vi "Monitor Tool Page.vi"(8 "error in (no error)":errorcluster, 11 "Node Ptr":T1 format="%.0x") -> (0 "error out":errorcluster)   [LabVIEW 2023, in "J1939 Addon System Explorer.lvlib"]
uses:
  J1939 Addon System Explorer.lvlib
  <vilib>/NI VeriStand/Custom Device API/Custom Device Item Ref.ctl
  Addon Shared/SubVIs/Constants.vi
  <vilib>/NI VeriStand/Custom Device API/Custom Device API.lvlib
  Addon Shared/J1939 Addon Shared.lvlib
panel:
  in  "Force SA":bool
  in  "Include DA":bool
  in  "Settings":cluster{"Section Name":string}={"Section Name"="J1939 Monitor Tool Settings"}
  in  "J1939 Name":u64 format="%.0x"
  in  "J1939 Network Address":u8 format="%.0x"
  in  "SHDocVw.IWebBrowser2":refnum<k7>(container)
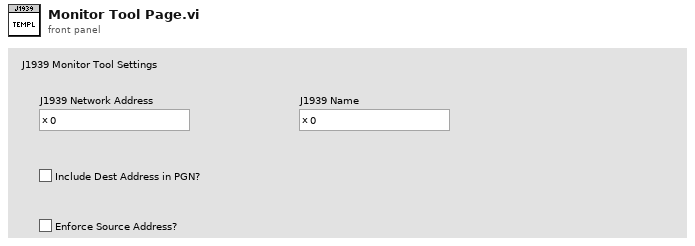
[diagram p1: front panel]
types:
  T1 = typedef "Custom Device API.lvlib/Custom Device Item Ref.ctl" = u64
  T2 = typedef "J1939 Addon Shared.lvlib/Monitor Settings.ctl" = cluster{"Address":u8, "Name":u64, "Include DA":bool, "Force SA":bool}
  T3 = typedef "Custom Device API.lvlib/Custom Device Commands.ctl" = enum16{"Default", "Item renamed", "Shutdown", "Dynamic button pressed"}
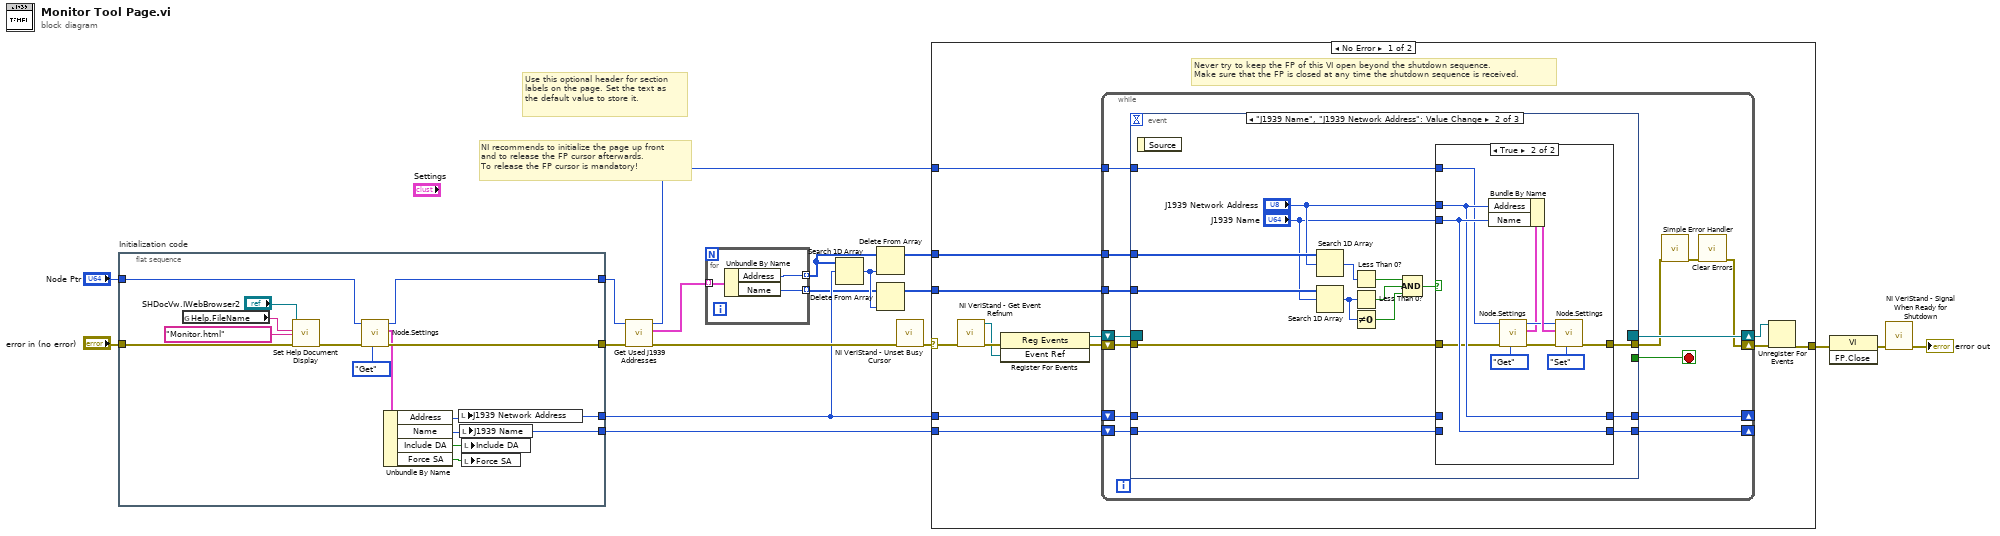
[diagram p0: block diagram]
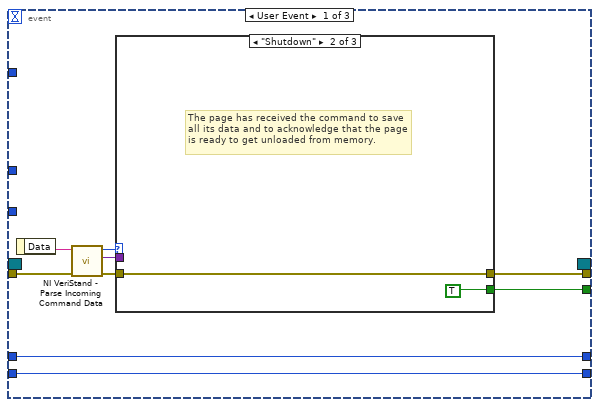
[diagram p2: hidden frame]
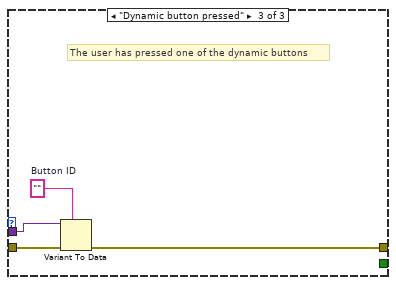
[diagram p4: hidden frame]
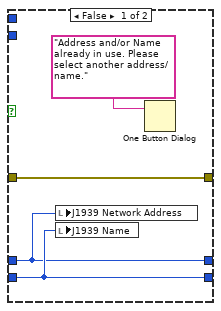
[diagram p5: hidden frame]
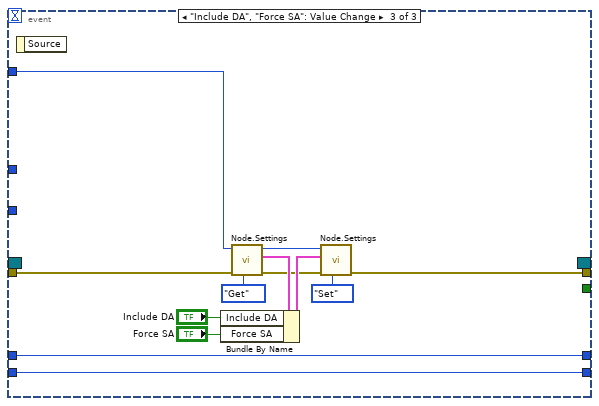
[diagram p6: hidden frame]
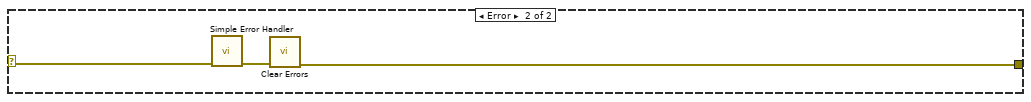
[diagram p7: hidden frame]
diagram:
  # "Use this optional header for section labels on the page. Set the text as the default value to store it."
  # "NI recommends to initialize the page up front\nand to release the FP cursor afterwards.\nTo release the FP cursor is mandatory!"
  n1 = flat-sequence "Initialization code" {
    tunnel: "error in (no error)" -> [w30]
    tunnel: "Node Ptr" -> [w27]
    tunnel: [w25] -> w11
    tunnel: [w23] -> w9
    tunnel: [w29] -> w7
    tunnel: [w28] -> w6
    frame #0 {
      n2 = global read "Constants.vi" "Help.FileName"() -> (w20:string)
      n3 = call "Set Help Document Display.vi"("error in (no error)"=w30, "HTML File"="Monitor.html", "Main CHM File"=w20, "SHDocVw.IWebBrowser2"="SHDocVw.IWebBrowser2") -> ("error out"=w26:errorcluster)  [unwired: 7 in]
      n4 = call "Node.Settings.vi"("Action"=enum8{"Get", "Set"}."Get", "error in (no error)"=w26, "Item Ref in"=w27) -> ("error out"=w25:errorcluster, "Node.Settings"=w24:T2, "Item Ref out"=w23:T1)  [unwired: 6 in]
      n5 = Unbundle By Name(w24) -> ("Address"=w29:u8, "Name"=w28:u64, "Include DA"=w21:bool, "Force SA"=w19:bool)
      n6 = local write "J1939 Network Address"(w29) -> ()
      n7 = local write "J1939 Name"(w28) -> ()
      n8 = local write "Include DA"(w21) -> ()
      n9 = local write "Force SA"(w19) -> ()
    }
  }
  n10 = call "Get Used J1939 Addresses.vi"("error in (no error)"=w11, "Node Ptr"=w9) -> ("error out"=w12:errorcluster, "Nodes"=w5:T2[], "Item Ref out"=w10:T1)  [unwired: 7 in]
  n11 = for {
    tunnel: w5 -> [w35] mode=indexing
    tunnel: [w34] -> w4 mode=indexing
    tunnel: [w33] -> w2 mode=indexing
    n12 = Unbundle By Name(w35) -> ("Address"=w34:u8, "Name"=w33:u64)
  }
  n13 = Search 1D Array(1D array=w4, element=w7) -> (index of element=w3:i32)  [unwired: 1 in]
  n14 = Delete From Array(array=w4, index=w3) -> (array with subset deleted=w8:u8[])  [unwired: 1 in, 1 out]
  n15 = Delete From Array(array=w2, index=w3) -> (array with subset deleted=w1:u64[])  [unwired: 1 in, 1 out]
  n16 = call <vilib>:"NI VeriStand - Unset Busy Cursor.vi"("error in (no error)"=w12) -> ("error out"=w14:errorcluster)  [unwired: 10 out]
  n17 = case shown="No Error" w14 {
    selector: w14 -> [w40 w126]
    tunnel: [w45 w124] -> w18
    tunnel: w10 -> [w41 _]
    tunnel: w8 -> [w39 _]
    tunnel: w7 -> [w38 _]
    tunnel: w6 -> [w37 _]
    tunnel: w1 -> [w36 _]
    frame No Error {
      # "Never try to keep the FP of this VI open beyond the shutdown sequence.\nMake sure that the FP is closed at any time the shutdown sequence is received."
      n18 = call <vilib>:"NI VeriStand - Get Event Refnum.vi"("error in (no error)"=w40) -> ("error out"=w48:errorcluster, "Event Ref"=w44:refnum<user-event>)  [unwired: 9 out]
      n19 = register-events(error in=w48, w44) -> (reference out=w42:refnum<event-registration>, error out=w43:errorcluster)  [unwired: 1 in]
      n20 = while {
        tunnel: w41 -> [w58]
        shift-right: [w55] -> w46
        shift-left: w43 -> [w61]
        shift-right: [w62] -> w47
        shift-left: w42 -> [w60]
        tunnel: w39 -> [w54]
        tunnel: w36 -> [w51]
        shift-right: [w49] -> _
        shift-left: w38 -> [w53]
        shift-right: [w50] -> _
        shift-left: w37 -> [w52]
        stop <- w59 stop-if-true
        n21 = event shown="[1] \"J1939 Name\", \"J1939 Network Address\": Value Change" {
          selector: w60 -> [_ _ _]
          dyn-events: [_ _ _] -> w62
          timeout: _ -> [_ _ _]
          tunnel: w61 -> [w71 w94 w117]
          tunnel: [w67 _ _] -> w59
          tunnel: [w66 w93 w123] -> w57
          tunnel: w58 -> [_ w95 w114]
          tunnel: w54 -> [_ w92 _]
          tunnel: w53 -> [w63 w90 w119]
          tunnel: w52 -> [w64 w89 w120]
          tunnel: w51 -> [_ w88 _]
          tunnel: [w64 w80 w120] -> w50
          tunnel: [w63 w79 w119] -> w49
          event User Event {
            n22 = event-data() -> ("Data"=w70:string)  [unwired: 1 out]
            n23 = call <vilib>:"NI VeriStand - Parse Incoming Command Data.vi"("error in (no error)"=w71, "Incoming data"=w70) -> ("error out"=w69:errorcluster, "Outgoing data"=w65:variant, "Action"=w68:T3)  [unwired: 7 out]
            n24 = case shown="\"Shutdown\"" w68 {
              tunnel: w69 -> [w72 w73 w78]
              tunnel: [_ TRUE _] -> w67
              tunnel: [w72 w73 w75] -> w66
              tunnel: w65 -> [_ _ w77]
              frame "Default", Default {
              }
              frame "Shutdown" {
                # "The page has received the command to save all its data and to acknowledge that the page is ready to get unloaded from memory."
              }
              frame "Dynamic button pressed" {
                w76 = ""  # Button ID
                # "The user has pressed one of the dynamic buttons"
                n25 = Variant To Data(error in=w78, type=w76, Variant=w77) -> (error out=w75:errorcluster)  [unwired: 1 out]
              }
            }
          }
          event "J1939 Name", "J1939 Network Address": Value Change {
            n26 = event-data() -> ()  [unwired: 2 out]
            n27 = Search 1D Array(1D array=w92, element="J1939 Network Address") -> (index of element=w84:i32)  [unwired: 1 in]
            n28 = Search 1D Array(1D array=w88, element="J1939 Name") -> (index of element=w82:i32)  [unwired: 1 in]
            n29 = Less Than 0?(x=w84) -> (x < 0?=w86:bool)
            n30 = Less Than 0?(x=w82) -> (x < 0?=w85:bool)
            n31 = Not Equal To 0?(x=w82) -> (x != 0?=w81:bool)
            n32 = Compound Arithmetic op=AND(w86, w85, w81) -> (w83:bool)
            n33 = case shown="True" w83 {
              tunnel: w95 -> [_ w102]
              tunnel: w94 -> [w99 w104]
              tunnel: [w99 w110] -> w93
              tunnel: "J1939 Network Address" -> [_ w108]
              tunnel: "J1939 Name" -> [_ w109]
              tunnel: w90 -> [w96 _]
              tunnel: w89 -> [w97 _]
              tunnel: [w97 w109] -> w80
              tunnel: [w96 w108] -> w79
              frame False {
                n34 = local write "J1939 Network Address"(w96) -> ()
                n35 = local write "J1939 Name"(w97) -> ()
                n36 = One Button Dialog(message="Address and/or Name already in use. Please select another address/name.") -> ()  [unwired: 1 in, 1 out]
              }
              frame True {
                n37 = call "Node.Settings.vi"("Action"=enum8{"Get", "Set"}."Get", "error in (no error)"=w104, "Item Ref in"=w102) -> ("error out"=w103:errorcluster, "Node.Settings"=w100:T2, "Item Ref out"=w101:T1)  [unwired: 6 in]
                n38 = Bundle By Name(cluster=w100, "Address"=w108, "Name"=w109) -> (w107:T2)
                n39 = call "Node.Settings.vi"("Action"=enum8{"Get", "Set"}."Set", "error in (no error)"=w103, "Node.Settings"=w107, "Item Ref in"=w101) -> ("error out"=w110:errorcluster)  [unwired: 5 in, 2 out]
              }
            }
          }
          event "Include DA", "Force SA": Value Change {
            n40 = event-data() -> ()  [unwired: 2 out]
            n41 = call "Node.Settings.vi"("Action"=enum8{"Get", "Set"}."Get", "error in (no error)"=w117, "Item Ref in"=w114) -> ("error out"=w115:errorcluster, "Node.Settings"=w116:T2, "Item Ref out"=w113:T1)  [unwired: 6 in]
            n42 = Bundle By Name(cluster=w116, "Include DA"="Include DA", "Force SA"="Force SA") -> (w122:T2)
            n43 = call "Node.Settings.vi"("Action"=enum8{"Get", "Set"}."Set", "error in (no error)"=w115, "Node.Settings"=w122, "Item Ref in"=w113) -> ("error out"=w123:errorcluster)  [unwired: 5 in, 2 out]
          }
        }
        n44 = call <vilib>:"Simple Error Handler.vi"("error in (no error)"=w57) -> ("error out"=w56:errorcluster)  [unwired: 1 in, 7 out]
        n45 = call <vilib>:"Clear Errors.vi"("error in (no error)"=w56) -> ("error out"=w55:errorcluster)  [unwired: 1 in, 5 out]
      }
      n46 = Unregister For Events(event registration refnum=w47, error in=w46) -> (error out=w45:errorcluster)
    }
    frame Error {
      n47 = call <vilib>:"Simple Error Handler.vi"("error in (no error)"=w126) -> ("error out"=w125:errorcluster)  [unwired: 1 in, 7 out]
      n48 = call <vilib>:"Clear Errors.vi"("error in (no error)"=w125) -> ("error out"=w124:errorcluster)  [unwired: 1 in, 5 out]
    }
  }
  n49 = invoke class="VI" method="FP.Close"(error in=w18) -> (error out=w17:errorcluster)  [unwired: 2 in, 2 out]
  n50 = call <vilib>:"NI VeriStand - Signal When Ready for Shutdown.vi"("error in (no error)"=w17) -> ("error out"=→"error out":errorcluster)  [unwired: 10 out]
